vi "load_config_v4_svi.vi"(8 "Config Directory":path) -> (2 "BETWEEN_PAT":u32, 3 "NPAT":u32, 4 "shoot_DURATION":dbl, 5 "shoot_at_SCAN":u32, 6 "is_single_shoot":bool, 7 "useLASER":bool, 9 "MIN_SCAN_DUR":dbl, 10 "Noff_fluidics":u32, 11 "BETEWEEN_SCAN":u32, 12 "USED_FILTERS 2":u8[](array[numeric]), 13 "Nstart_laser":u32, 14 "USED_LEDS 2":bool[][](array[boolean]), 15 "NSCAN":u32, 16 "EXPT":dbl, 17 "Non_laser":u32, 18 "Non_fluidics":u32, 19 "XYPOS":T1 caption="XYPOS 2", 20 "Refnum VISA en sortie":refnum<visa-resource-name>, 21 "BIN":u16, 22 "Nstart_fluidics":u32, 23 "ROMODE":u32, 24 "useFLUIDICS":bool, 25 "STAGE_SPEED":dbl, 26 "Noff_laser":u32)   [LabVIEW 2013]
uses:
  <vilib>/Analysis/Matrix/Datatypes/RealMatrix.ctl
  <vilib>/Analysis/Matrix/NI_Matrix.lvlib
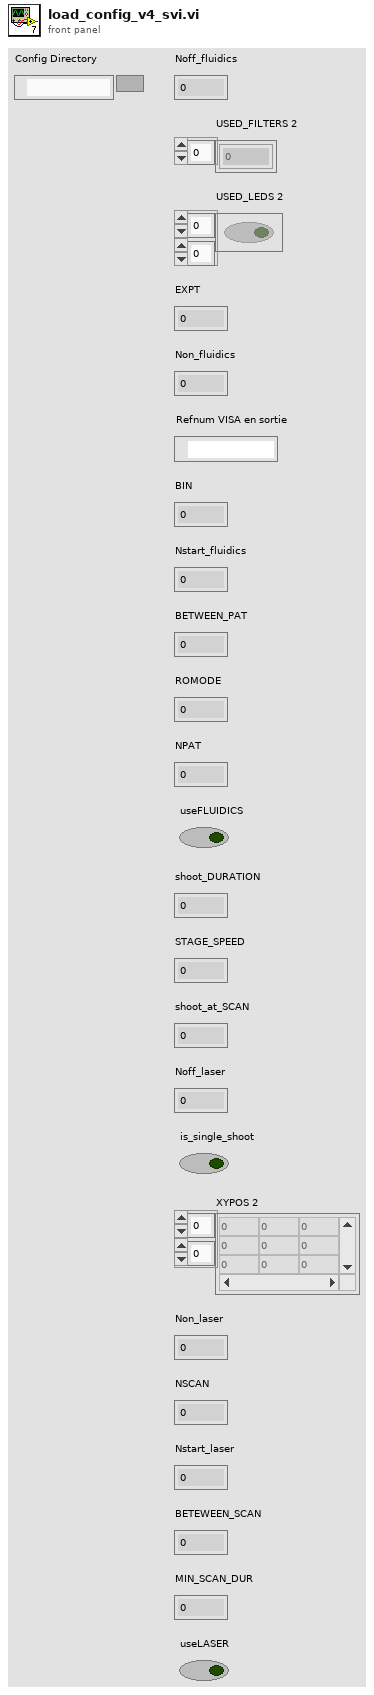
[diagram p1: front panel]
types:
  T1 = typedef "NI_Matrix.lvlib/RealMatrix.ctl" = dbl[][]
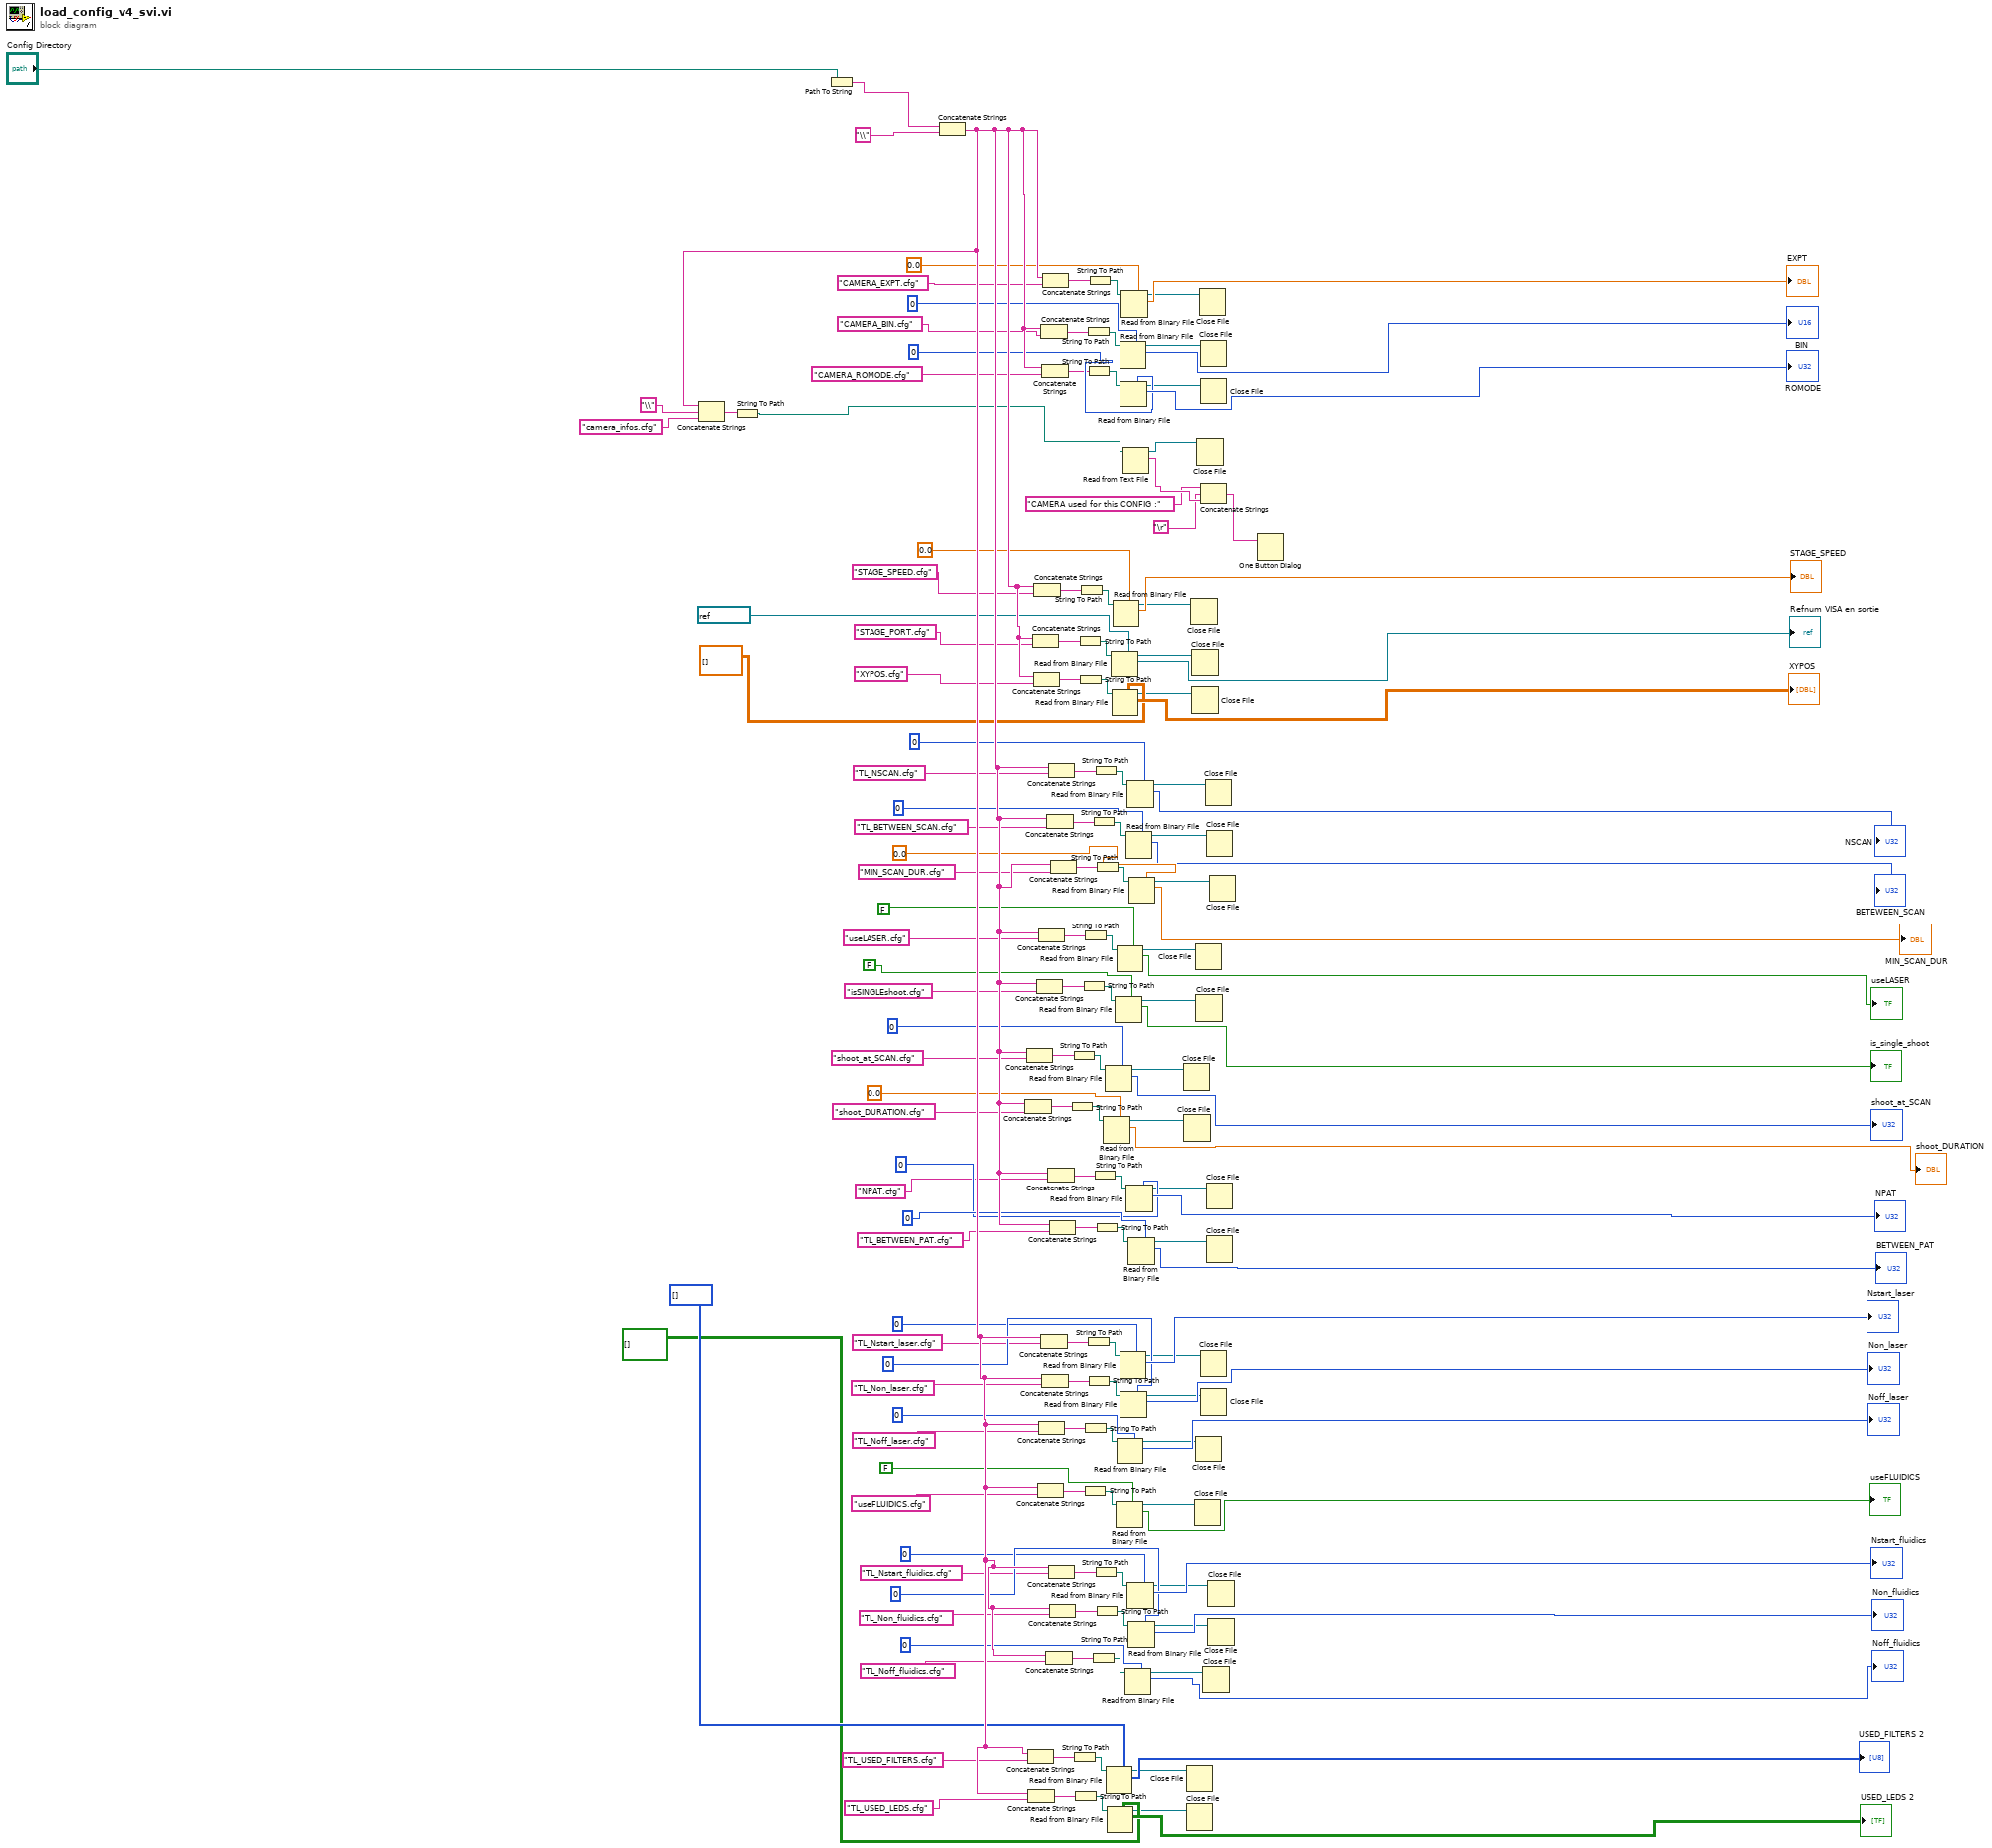
[diagram p0: block diagram]
diagram:
  n1 = Path To String(path="Config Directory") -> (string=w66:string)
  n2 = Concatenate Strings(w66, "\\") -> (w157:string)
  n3 = Concatenate Strings(w157, "\\", "camera_infos.cfg") -> (w63:string)
  n4 = String To Path(string=w63) -> (path=w67:path)
  n5 = Concatenate Strings(w157, "shoot_DURATION.cfg") -> (w112:string)
  n6 = Concatenate Strings(w157, "shoot_at_SCAN.cfg") -> (w111:string)
  n7 = Concatenate Strings(w157, "TL_USED_FILTERS.cfg") -> (w46:string)
  n8 = Concatenate Strings(w157, "TL_USED_LEDS.cfg") -> (w47:string)
  n9 = Concatenate Strings(w157, "STAGE_PORT.cfg") -> (w16:string)
  n10 = Concatenate Strings(w157, "XYPOS.cfg") -> (w17:string)
  n11 = Concatenate Strings(w157, "STAGE_SPEED.cfg") -> (w15:string)
  n12 = Concatenate Strings(w157, "isSINGLEshoot.cfg") -> (w104:string)
  n13 = Concatenate Strings(w157, "useFLUIDICS.cfg") -> (w148:string)
  n14 = Concatenate Strings(w157, "useLASER.cfg") -> (w103:string)
  n15 = Concatenate Strings(w157, "TL_Noff_laser.cfg") -> (w45:string)
  n16 = Concatenate Strings(w157, "CAMERA_BIN.cfg") -> (w6:string)
  n17 = Concatenate Strings(w157, "TL_Nstart_laser.cfg") -> (w37:string)
  n18 = Concatenate Strings(w157, "CAMERA_ROMODE.cfg") -> (w10:string)
  n19 = Concatenate Strings(w157, "TL_Non_laser.cfg") -> (w38:string)
  n20 = Concatenate Strings(w157, "CAMERA_EXPT.cfg") -> (w5:string)
  n21 = Concatenate Strings(w157, "TL_Noff_fluidics.cfg") -> (w133:string)
  n22 = Concatenate Strings(w157, "TL_BETWEEN_SCAN.cfg") -> (w28:string)
  n23 = Concatenate Strings(w157, "NPAT.cfg") -> (w29:string)
  n24 = Concatenate Strings(w157, "TL_NSCAN.cfg") -> (w27:string)
  n25 = Concatenate Strings(w157, "TL_Nstart_fluidics.cfg") -> (w127:string)
  n26 = Concatenate Strings(w157, "TL_BETWEEN_PAT.cfg") -> (w36:string)
  n27 = Concatenate Strings(w157, "TL_Non_fluidics.cfg") -> (w128:string)
  n28 = Concatenate Strings(w157, "MIN_SCAN_DUR.cfg") -> (w151:string)
  n29 = String To Path(string=w112) -> (path=w114:path)
  n30 = String To Path(string=w111) -> (path=w113:path)
  n31 = String To Path(string=w46) -> (path=w49:path)
  n32 = String To Path(string=w47) -> (path=w50:path)
  n33 = String To Path(string=w16) -> (path=w19:path)
  n34 = String To Path(string=w17) -> (path=w20:path)
  n35 = String To Path(string=w15) -> (path=w18:path)
  n36 = String To Path(string=w104) -> (path=w106:path)
  n37 = String To Path(string=w148) -> (path=w145:path)
  n38 = String To Path(string=w103) -> (path=w105:path)
  n39 = String To Path(string=w45) -> (path=w48:path)
  n40 = String To Path(string=w6) -> (path=w7:path)
  n41 = String To Path(string=w37) -> (path=w40:path)
  n42 = String To Path(string=w10) -> (path=w11:path)
  n43 = String To Path(string=w38) -> (path=w41:path)
  n44 = String To Path(string=w5) -> (path=w3:path)
  n45 = String To Path(string=w133) -> (path=w134:path)
  n46 = String To Path(string=w28) -> (path=w31:path)
  n47 = String To Path(string=w29) -> (path=w32:path)
  n48 = String To Path(string=w27) -> (path=w30:path)
  n49 = String To Path(string=w127) -> (path=w129:path)
  n50 = String To Path(string=w36) -> (path=w39:path)
  n51 = String To Path(string=w128) -> (path=w130:path)
  n52 = String To Path(string=w151) -> (path=w152:path)
  n53 = Read from Binary File(5:0.0, 11:w114) -> (2:→"shoot_DURATION":dbl, 3:w116:refnum<file>)  [unwired: 4 in, 2 out]
  n54 = Read from Binary File(5:u32 0, 11:w113) -> (2:→"shoot_at_SCAN":u32, 3:w115:refnum<file>)  [unwired: 4 in, 2 out]
  n55 = Read from Binary File(5:u8[] [] ("USED_FILTERS 2"), 11:w49) -> (2:→"USED_FILTERS 2":u8[], 3:w52:refnum<file>)  [unwired: 4 in, 2 out]
  n56 = Read from Binary File(5:bool[][] [] ("USED_LEDS 2"), 11:w50) -> (2:→"USED_LEDS 2":bool[][], 3:w53:refnum<file>)  [unwired: 4 in, 2 out]
  n57 = Read from Binary File(5:refnum<visa-resource-name> "COM1" ("STAGE_PORT 2"), 11:w19) -> (2:→"Refnum VISA en sortie":refnum<visa-resource-name>, 3:w22:refnum<file>)  [unwired: 4 in, 2 out]
  n58 = Read from Binary File(5:T1 [] ("XYPOS 2"), 11:w20) -> (2:→"XYPOS":T1, 3:w23:refnum<file>)  [unwired: 4 in, 2 out]
  n59 = Read from Binary File(5:0.0, 11:w18) -> (2:→"STAGE_SPEED":dbl, 3:w21:refnum<file>)  [unwired: 4 in, 2 out]
  n60 = Read from Binary File(5:FALSE, 11:w106) -> (2:→"is_single_shoot":bool, 3:w108:refnum<file>)  [unwired: 4 in, 2 out]
  n61 = Read from Binary File(5:FALSE, 11:w145) -> (2:→"useFLUIDICS":bool, 3:w146:refnum<file>)  [unwired: 4 in, 2 out]
  n62 = Read from Binary File(5:FALSE, 11:w105) -> (2:→"useLASER":bool, 3:w107:refnum<file>)  [unwired: 4 in, 2 out]
  n63 = Read from Binary File(5:u32 0, 11:w48) -> (2:→"Noff_laser":u32, 3:w51:refnum<file>)  [unwired: 4 in, 2 out]
  n64 = Read from Binary File(5:u16 0, 11:w7) -> (2:→"BIN":u16, 3:w13:refnum<file>)  [unwired: 4 in, 2 out]
  n65 = Read from Binary File(5:u32 0, 11:w40) -> (2:→"Nstart_laser":u32, 3:w43:refnum<file>)  [unwired: 4 in, 2 out]
  n66 = Read from Binary File(5:u32 0, 11:w11) -> (2:→"ROMODE":u32, 3:w14:refnum<file>)  [unwired: 4 in, 2 out]
  n67 = Read from Binary File(5:u32 0, 11:w41) -> (2:→"Non_laser":u32, 3:w44:refnum<file>)  [unwired: 4 in, 2 out]
  n68 = Read from Binary File(5:0.0, 11:w3) -> (2:→"EXPT":dbl, 3:w12:refnum<file>)  [unwired: 4 in, 2 out]
  n69 = Read from Text File(file (use dialog)=w67) -> (refnum out=w68:refnum<file>, text=w71:string)  [unwired: 3 in, 2 out]
  n70 = Read from Binary File(5:u32 0, 11:w134) -> (2:→"Noff_fluidics":u32, 3:w135:refnum<file>)  [unwired: 4 in, 2 out]
  n71 = Read from Binary File(5:u32 0, 11:w31) -> (2:→"BETEWEEN_SCAN":u32, 3:w34:refnum<file>)  [unwired: 4 in, 2 out]
  n72 = Read from Binary File(5:u32 0, 11:w32) -> (2:→"NPAT":u32, 3:w35:refnum<file>)  [unwired: 4 in, 2 out]
  n73 = Read from Binary File(5:u32 0, 11:w30) -> (2:→"NSCAN":u32, 3:w33:refnum<file>)  [unwired: 4 in, 2 out]
  n74 = Read from Binary File(5:u32 0, 11:w129) -> (2:→"Nstart_fluidics":u32, 3:w131:refnum<file>)  [unwired: 4 in, 2 out]
  n75 = Read from Binary File(5:u32 0, 11:w39) -> (2:→"BETWEEN_PAT":u32, 3:w42:refnum<file>)  [unwired: 4 in, 2 out]
  n76 = Read from Binary File(5:u32 0, 11:w130) -> (2:→"Non_fluidics":u32, 3:w132:refnum<file>)  [unwired: 4 in, 2 out]
  n77 = Read from Binary File(5:0.0, 11:w152) -> (2:→"MIN_SCAN_DUR":dbl, 3:w153:refnum<file>)  [unwired: 4 in, 2 out]
  n78 = Close File(refnum=w115) -> ()  [unwired: 1 in, 2 out]
  n79 = Close File(refnum=w116) -> ()  [unwired: 1 in, 2 out]
  n80 = Close File(refnum=w52) -> ()  [unwired: 1 in, 2 out]
  n81 = Close File(refnum=w53) -> ()  [unwired: 1 in, 2 out]
  n82 = Close File(refnum=w21) -> ()  [unwired: 1 in, 2 out]
  n83 = Close File(refnum=w22) -> ()  [unwired: 1 in, 2 out]
  n84 = Close File(refnum=w23) -> ()  [unwired: 1 in, 2 out]
  n85 = Close File(refnum=w146) -> ()  [unwired: 1 in, 2 out]
  n86 = Close File(refnum=w107) -> ()  [unwired: 1 in, 2 out]
  n87 = Close File(refnum=w51) -> ()  [unwired: 1 in, 2 out]
  n88 = Close File(refnum=w108) -> ()  [unwired: 1 in, 2 out]
  n89 = Close File(refnum=w68) -> ()  [unwired: 1 in, 2 out]
  n90 = Close File(refnum=w12) -> ()  [unwired: 1 in, 2 out]
  n91 = Close File(refnum=w13) -> ()  [unwired: 1 in, 2 out]
  n92 = Close File(refnum=w14) -> ()  [unwired: 1 in, 2 out]
  n93 = Concatenate Strings("CAMERA used for this CONFIG :", "\r", w71) -> (w72:string)
  n94 = Close File(refnum=w43) -> ()  [unwired: 1 in, 2 out]
  n95 = Close File(refnum=w44) -> ()  [unwired: 1 in, 2 out]
  n96 = Close File(refnum=w135) -> ()  [unwired: 1 in, 2 out]
  n97 = Close File(refnum=w33) -> ()  [unwired: 1 in, 2 out]
  n98 = Close File(refnum=w34) -> ()  [unwired: 1 in, 2 out]
  n99 = Close File(refnum=w35) -> ()  [unwired: 1 in, 2 out]
  n100 = Close File(refnum=w42) -> ()  [unwired: 1 in, 2 out]
  n101 = Close File(refnum=w131) -> ()  [unwired: 1 in, 2 out]
  n102 = Close File(refnum=w132) -> ()  [unwired: 1 in, 2 out]
  n103 = Close File(refnum=w153) -> ()  [unwired: 1 in, 2 out]
  n104 = One Button Dialog(message=w72) -> ()  [unwired: 1 in, 1 out]
